vi "PDF_Interface_PDF Protokoll CalGas.vi"(8 "error in (no error)":errorcluster caption="Fehler (Eingang, kein Fehler)", 10 "Save PDF File Path":path, 11 "Zeitstempel":timestamp) -> (0 "error out":errorcluster caption="Fehler (Ausgang)")   [LabVIEW 2020, in "Erweiterte Konfig.lvlib" / "CG-Check Konfig.lvlib"]
uses:
  CG-Check Konfig.lvlib
  Sprachverwaltung/FGV Aktion Tabelle zerlegen.ctl
  System Einstellungen V2/Aktioen FGV System Konstanten.ctl
  Aktion_CG-Check.ctl
  Schedule Modul/Aktion FGV Testdaten sammeln.ctl
  FT-IR/FGV FT-IR Gasliste Aktionen.ctl
  Gaszuordnung AO/FGV Gaszuordnung Grenzen&Einheit Aktion.ctl
  PDF_Interface/PDF Protokoll Standard Kopf Optionen.ctl
  <vilib>/Simplicity AI/SAI_PDF_API/Classes/Context/Controls/SAI_PDF_PDF Details.ctl
  PDF_Interface/PDF Interface Helper/PDFContentType.ctl
  PDF_Interface/PDF Interface Helper/PDFTableContentType.ctl
  PDF_Interface/PDF Interface Helper/PDFResults.ctl
  PDF_Interface/PDF Interface Helper/PDFResultPictures.ctl
  PDF_Interface/PDF Interface Helper/PDFCommentPosition.ctl
  PDF_Interface/PDF Interface Helper/PDFPageBreak.ctl
  PDF_Interface/PDF Interface Helper/PDFTablePictures.ctl
  PDF_Interface/PDF Interface Helper/PDFBemerkung.ctl
  <vilib>/Simplicity AI/SAI_PDF_API/Classes/Context/Controls/SAI_PDF_Text Align.ctl
  <vilib>/Simplicity AI/SAI_PDF_API/Classes/Context/Controls/SAI_PDF_Font.ctl
  <vilib>/Simplicity AI/SAI_PDF_API/Classes/Context/Controls/SAI_PDF_Font Encoding.ctl
  Schedule Modul/Schedule Modul.lvlib
  System Einstellungen V2/System Einstellungen V2.lvlib
  FT-IR/FT-IR.lvlib
  Gaszuordnung AO/Gaszuordnung AO.lvlib
  Allgemein/allgemeine Sub-VIs.lvlib
  Sprachverwaltung/Sprachverwaltung.lvlib
  Linearisierung V2/Protokoll/Protokoll.lvlib
  PDF_Interface/PDF Interface.lvlib
  <vilib>/Simplicity AI/SAI_PDF_API/Classes/Context/Context.lvclass
  PDF_Interface/PDF Interface Helper/PDF Interface Helper.lvlib
panel:
  out "Span Eingang 3":string[][](table)
  out "Ergebnis 3":string caption="Auswertung:"
  out "Span Eingang 2":string[][](table)
  out "Ergebnis 2":string caption="Auswertung:"
  out "Span Eingang 1":string[][](table)
  out "Ergebnis":string caption="Auswertung:"
  out "Datum":string caption="Datum:"
  out "Messgerät:":string
  # "Kalibriergastest Protokoll"
  # "Ergebnisse:"
  # "IAG-Industrie Automatisierungsgeschellschaft m.b.H.    l  Industriestraße 322    l    2722Weikersdorf     )+43262241712/0"
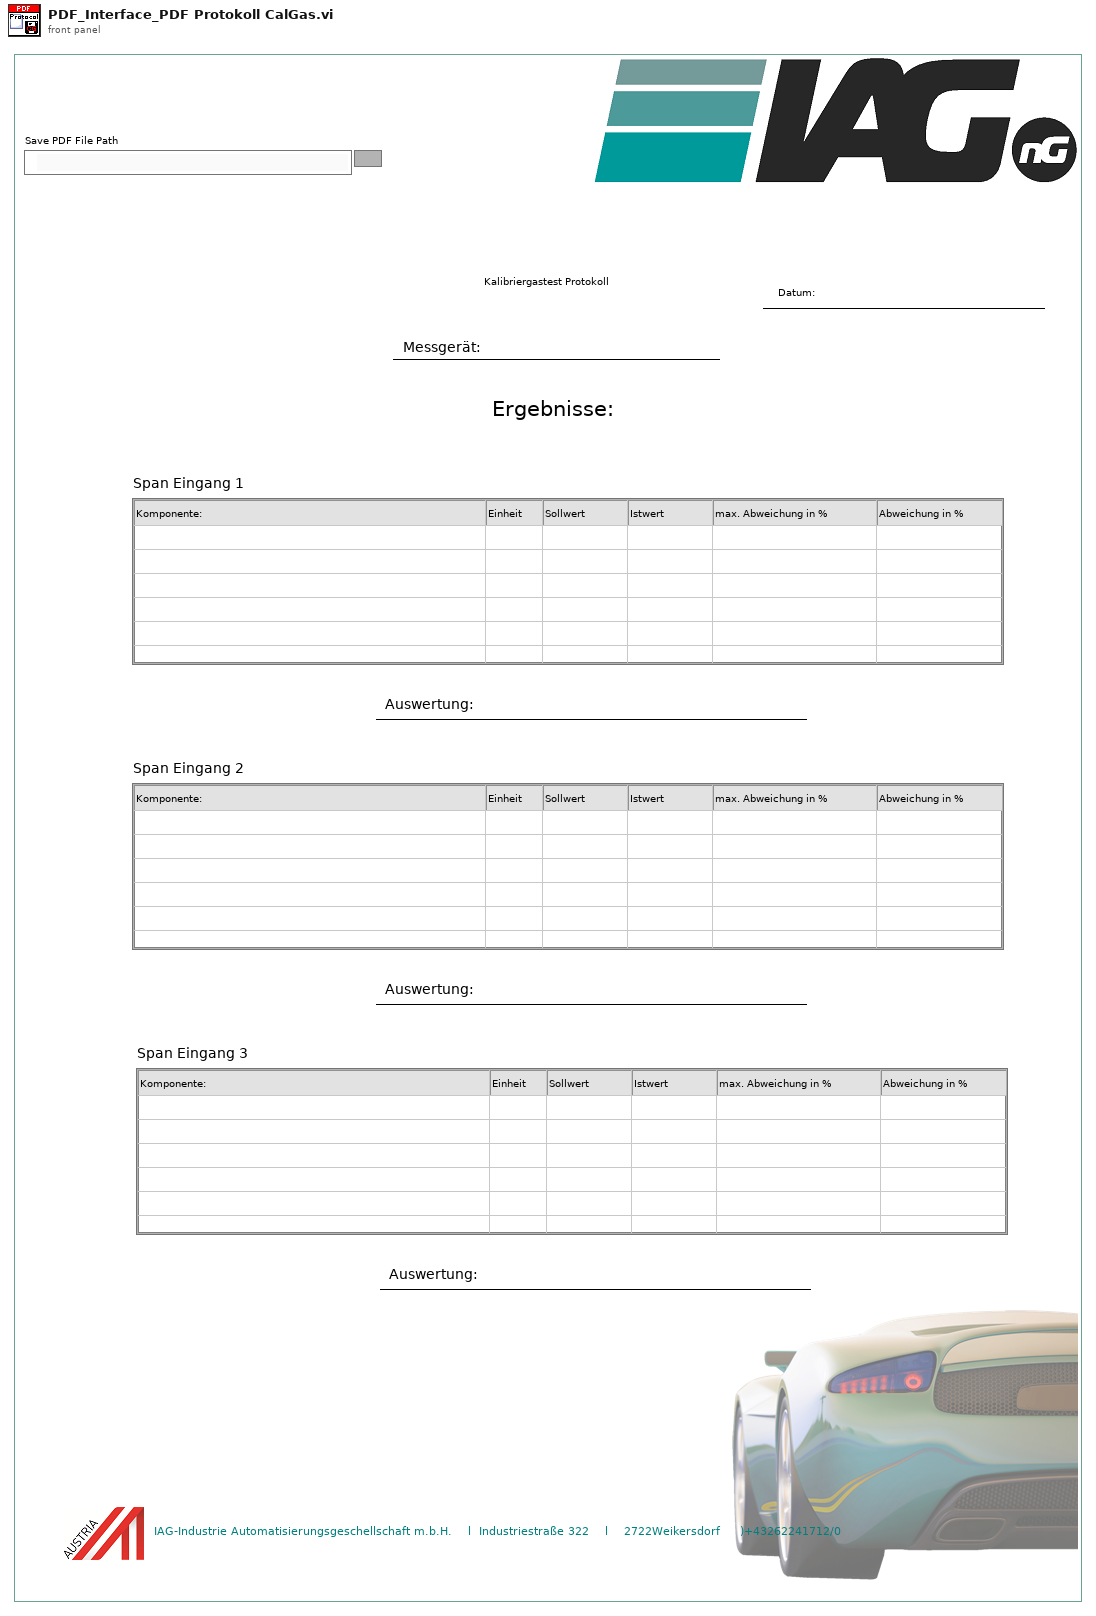
[diagram p1: front panel]
types:
  T1 = typedef "Sprachverwaltung.lvlib/FGV Aktion Tabelle zerlegen.ctl" = enum16{"laden", "vereinzeln", "speichern"}
  T2 = typedef "Schedule Modul.lvlib/Aktion FGV Testdaten sammeln.ctl" = enum16{"lesen", "Dichtheitstest", "CalGasTest", "T90", "Kalibrieren", "init", "Kalender Daten"}
  T3 = typedef "Erweiterte Konfig.lvlib/CG-Check Konfig.lvlib/Aktion_CG-Check.ctl" = enum16{"lesen", "schreiben", "laden", "Komponente", "Aktive?", "speichern"}
  T4 = typedef "System Einstellungen V2.lvlib/Aktioen FGV System Konstanten.ctl" = enum16{"lesen", "laden", "speichern", "Sprache"}
  T5 = typedef "FT-IR.lvlib/FGV FT-IR Gasliste Aktionen.ctl" = enum16{"lesen", "Gasliste FT-IR", "Gasliste ausgelesen", "laden", "speichern", "löschen"}
  T6 = typedef "Gaszuordnung AO.lvlib/FGV Gaszuordnung Grenzen&Einheit Aktion.ctl" = enum16{"Lesen", "Schreiben Min", "Schreiben Max", "Laden", "Speichern"}
  T7 = typedef "PDF Interface.lvlib/PDF Interface Helper.lvlib/PDFTableContentType.ctl" = cluster{"TableHeader":string[], "Table":string[][], "Relative Column Widths (%)":sgl[], "Results":T8, "PositionBemerkung":T10, "PageBreak":T11, "TablePictures":T12, "Horizontal Align":i32}
  T8 = typedef "PDF Interface.lvlib/PDF Interface Helper.lvlib/PDFResults.ctl" = cluster{"Results":cluster{"Result Text":string, "Result":bool}[], "ResultPictures":T9, "use Pictures":bool, "Image Scale (%)":sgl, "Autoscale? (T)":bool, "Horizontal Align":i32, "Position":i32}
  T9 = typedef "PDF Interface.lvlib/PDF Interface Helper.lvlib/PDFResultPictures.ctl" = cluster{"Yes Ctl Refnum":refnum<vi>, "No Ctl Refnum":refnum<vi>}
  T10 = typedef "PDF Interface.lvlib/PDF Interface Helper.lvlib/PDFCommentPosition.ctl" = enum16{"before", "after"}
  T11 = typedef "PDF Interface.lvlib/PDF Interface Helper.lvlib/PDFPageBreak.ctl" = enum16{"none", "before", "after", "after comment"}
  T12 = typedef "PDF Interface.lvlib/PDF Interface Helper.lvlib/PDFTablePictures.ctl" = cluster{"Ctl Refnum In":refnum<vi>[], "RowOrColumn":enum16{"Row", "Column"}, "IndexToInsert":u16, "Image Scale (%)":sgl[], "Autoscale? (T)":bool[], "Horizontal Align":i32}
  T13 = typedef "PDF Interface.lvlib/PDF Interface Helper.lvlib/PDFContentType.ctl" = cluster{"Titel":string, "Header Table":string[][], "Table Array":T7[], "Bemerkungen":T14[]}
  T14 = typedef "PDF Interface.lvlib/PDF Interface Helper.lvlib/PDFBemerkung.ctl" = cluster{"Bemerkung Text":string, "Align (Left)":T15, "Add Line Feeds (F:No)":bool, "Font":T16}
  T15 = typedef "SAI_PDF_Toolkit.lvlib/Context.lvclass/SAI_PDF_Text Align.ctl" = i32
  T16 = typedef "SAI_PDF_Toolkit.lvlib/Context.lvclass/SAI_PDF_Font.ctl" = cluster{"Font":string, "Size":i32, "Colour":u32, "Bold":bool, "Italic":bool, "Underline":bool, "Strikethrough":bool, "Font Encoding":T17}
  T17 = typedef "SAI_PDF_Toolkit.lvlib/Context.lvclass/SAI_PDF_Font Encoding.ctl" = enum16{"Cp1252, WinANSI", "IdentityH", "IdentityV", "Cp1250", "Cp1257", "MacRoman"}
  T18 = typedef "SAI_PDF_Toolkit.lvlib/Context.lvclass/SAI_PDF_PDF Details.ctl" = cluster{"Title":string, "Subject":string, "Keywords":string, "Author":string, "Creator":string}
  T19 = cluster{"Header Footer Text Cluster":cluster{"Header Text":string, "Footer Text":string, "Time":string, "Page Number":string}, "PDF Details":T18}
  T20 = typedef "PDF Interface.lvlib/PDF Protokoll Standard Kopf Optionen.ctl" = cluster{"Analysator":bool, "FT-IR Rezept":bool, "Gasteiler":bool, "Gas Komponente":bool, "Gas Flasche":bool, "LIN Protokoll":bool, "Operator":bool}
  T21 = typedef "Schedule Modul.lvlib/Ergebnis CalGas Test.ctl" = cluster{"Istwerte":string[][], "Auswertung":string[][][], "Fehler":bool[], "Abweichung in %":string[][], "Spanauswahl":i32[]}
  T22 = typedef "String - Ausgabefeld.ctl" = string
  T23 = cluster{"Modell":string, "ProjektNummer":string, "Software Version":string, "Seriennummer":string}
  T24 = cluster{"Header Size":i32, "Column Ratio left":sgl[]}
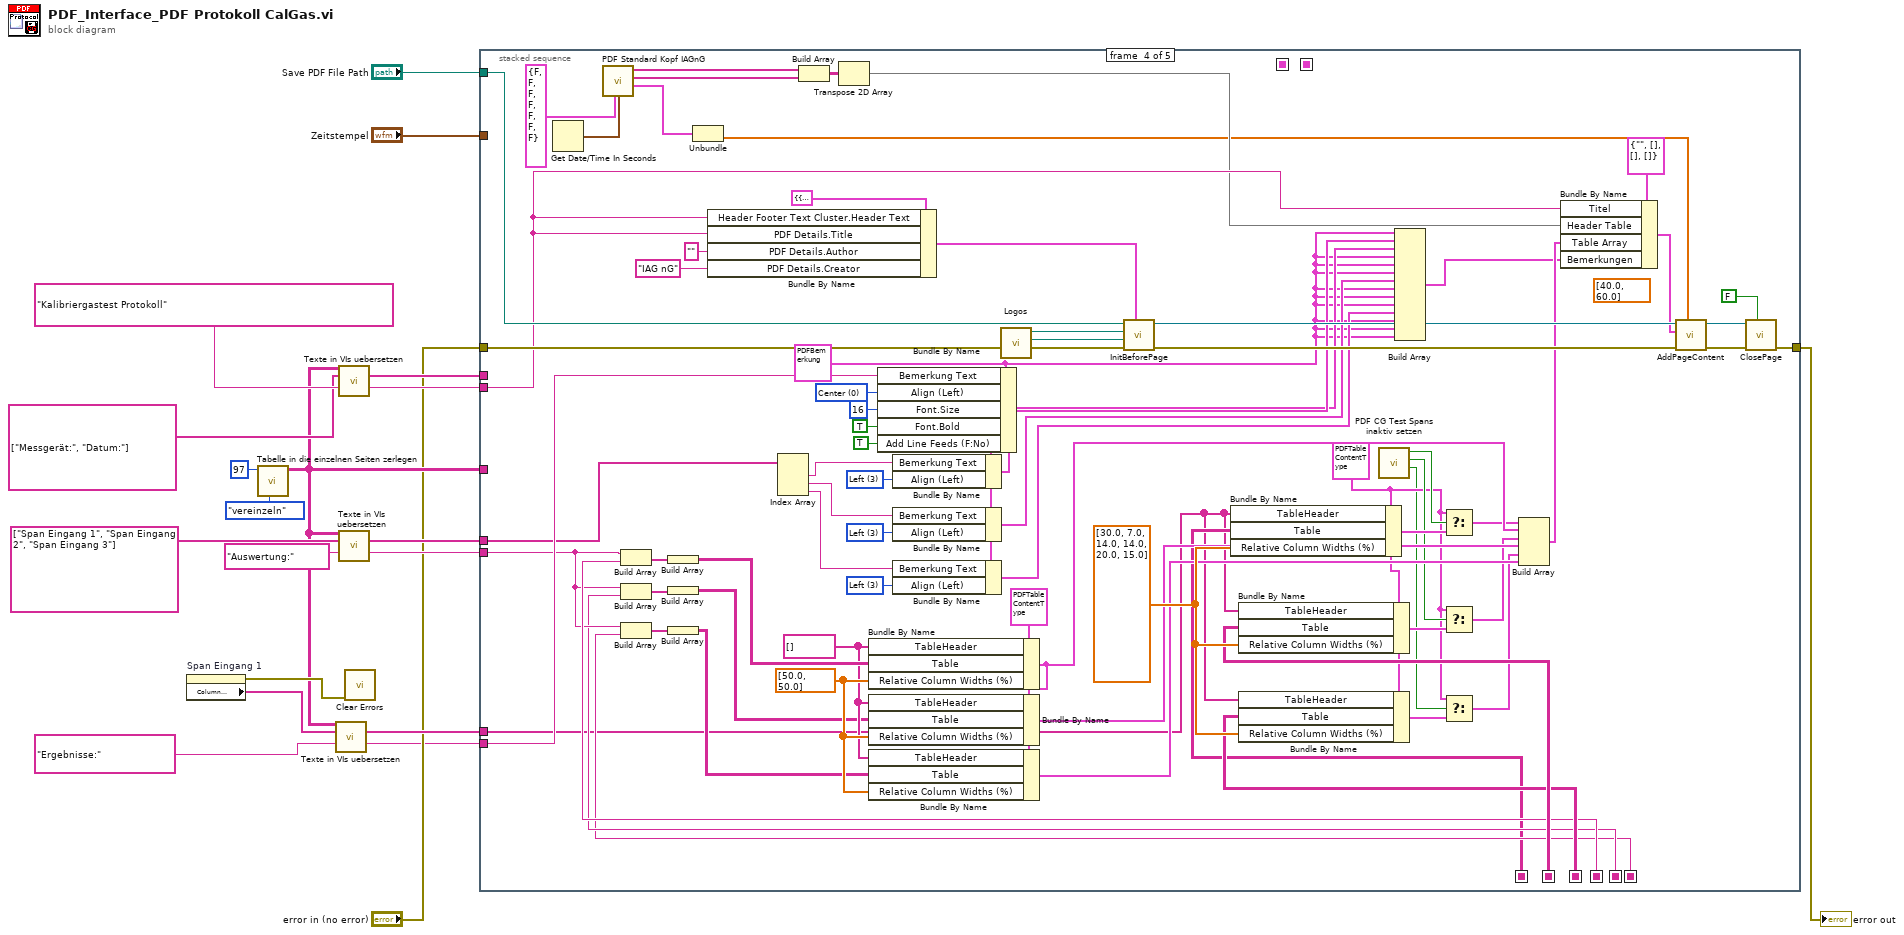
[diagram p0: block diagram]
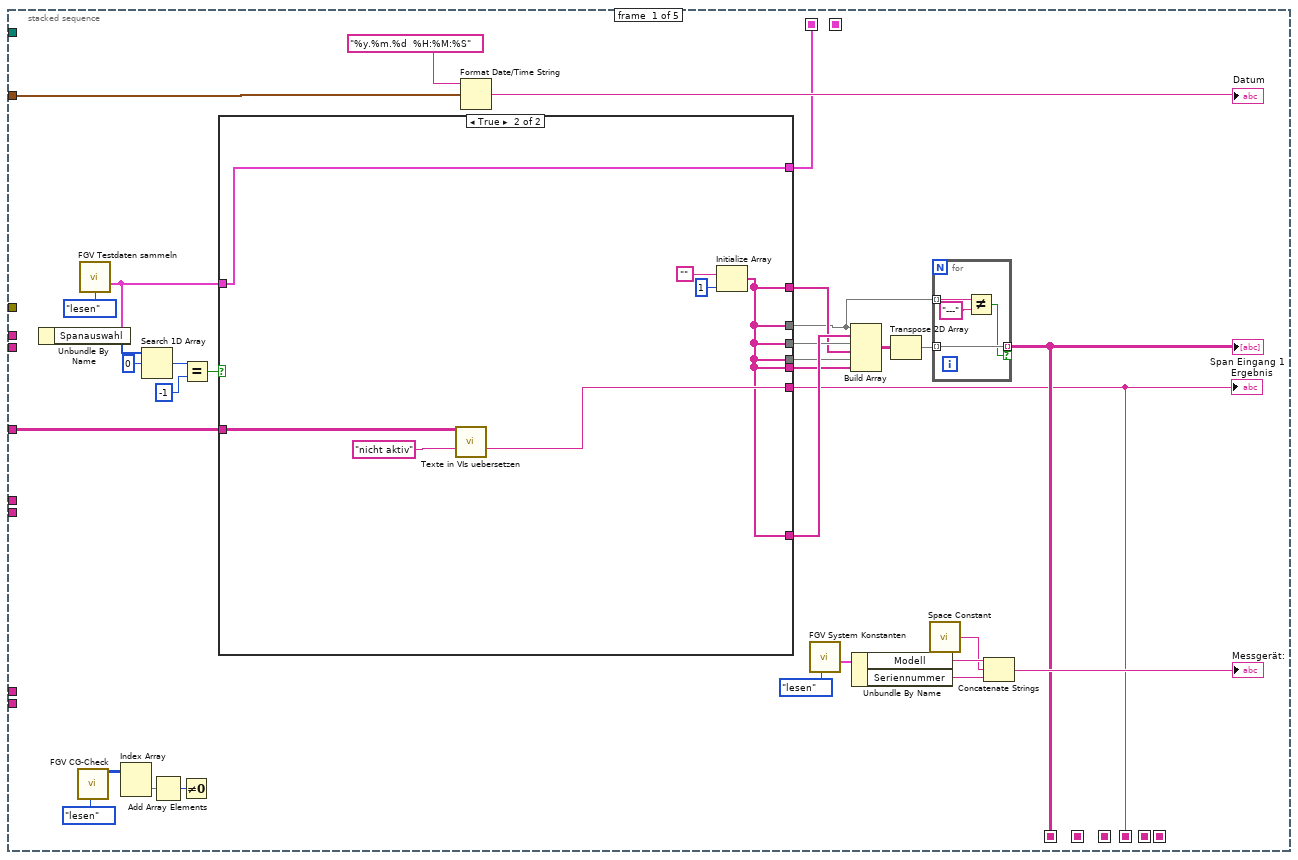
[diagram p2: hidden frame]
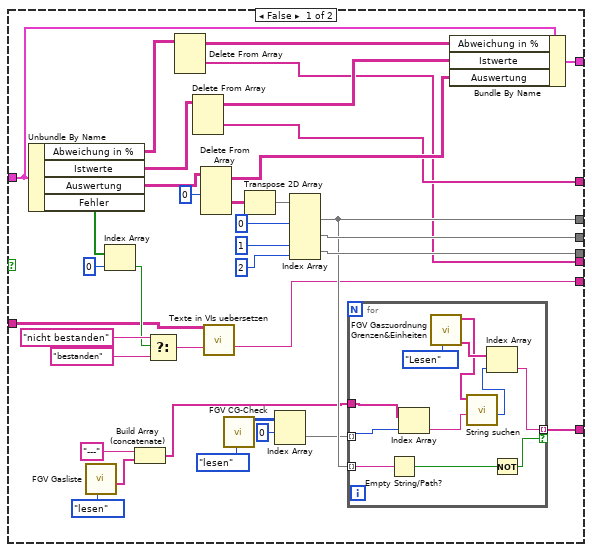
[diagram p3: hidden frame]
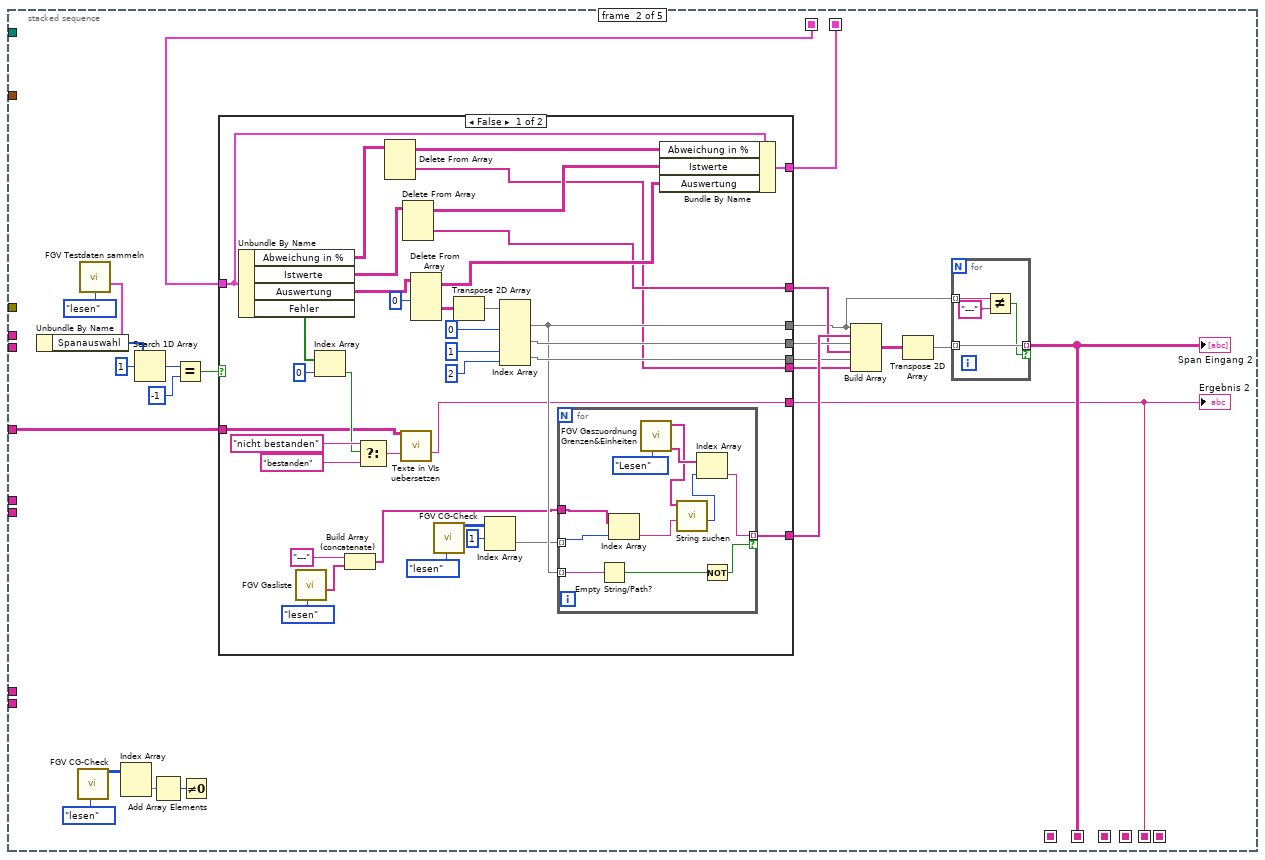
[diagram p4: hidden frame]
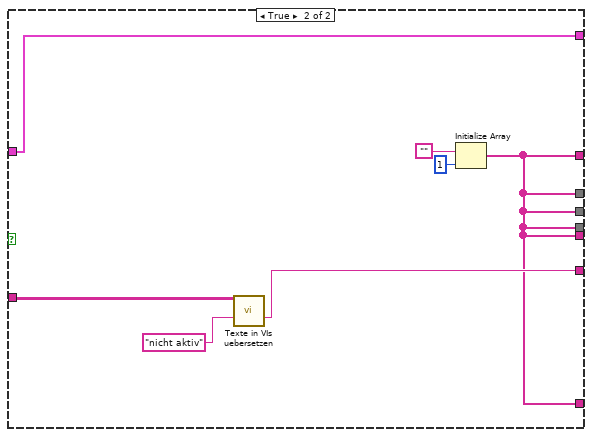
[diagram p5: hidden frame]
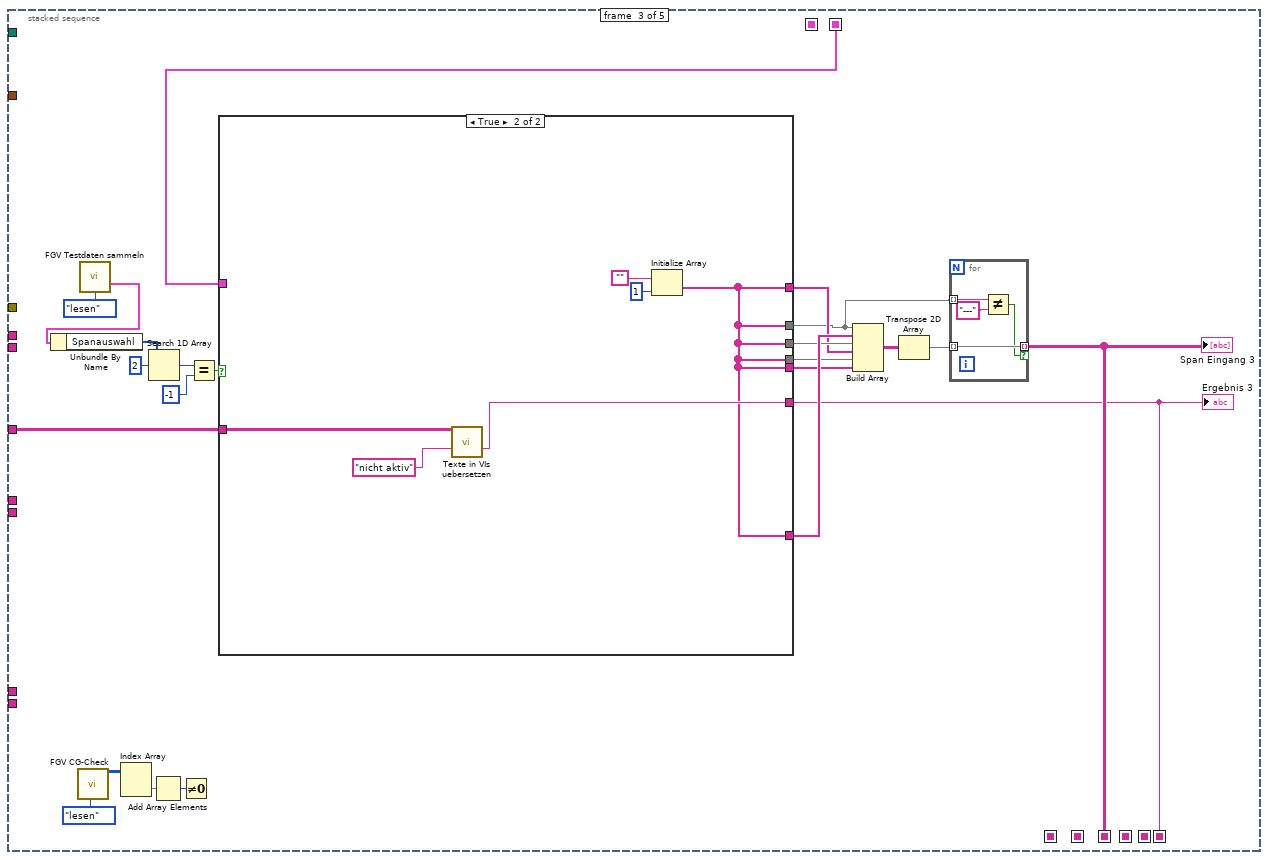
[diagram p6: hidden frame]
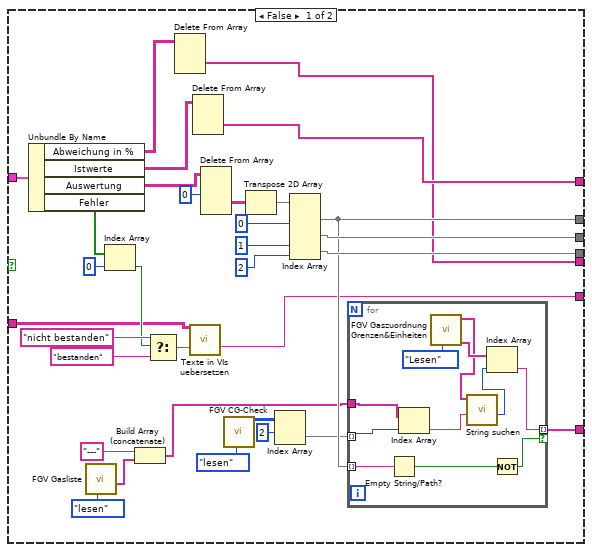
[diagram p7: hidden frame]
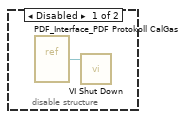
[diagram p9: hidden frame]
diagram:
  n1 = property on="Span Eingang 1" class="Tbl (strikt)"() -> (error out=w9:errorcluster, "Column Headers[]"=w8:string[])  [unwired: 2 in, 1 out]
  n2 = call "Tabelle in die einzelnen Seiten zerlegen.vi"("Aktion"=FGV_Aktion_Tabelle_zerlegen."vereinzeln", "Index (Seite)"=97) -> ("Sprachliste"=w7:string[][])  [unwired: 7 in, 2 out]
  n3 = call "Texte in VIs uebersetzen.vi"("Sprachliste"=w7, "String-Array zum Übersetzen"=w8, "String zum Übersetzen"="Ergebnisse:") -> ("String-Array zum Übersetzen"=w6:string[], "String zum Übersetzen"=w1:string)  [unwired: 8 in, 3 out]
  n4 = call "Texte in VIs uebersetzen.vi"("Sprachliste"=w7, "String-Array zum Übersetzen"=string[] ["Messgerät:", "Datum:"], "String zum Übersetzen"="Kalibriergastest Protokoll") -> ("String-Array zum Übersetzen"=w14:string[], "String zum Übersetzen"=w15:string)  [unwired: 8 in, 3 out]
  n5 = call "Texte in VIs uebersetzen.vi"("Sprachliste"=w7, "String-Array zum Übersetzen"=string[] ["Span Eingang 1", "Span Eingang 2", "Span Eingang 3"], "String zum Übersetzen"="Auswertung:") -> ("String-Array zum Übersetzen"=w12:string[], "String zum Übersetzen"=w10:string)  [unwired: 8 in, 3 out]
  n6 = call <vilib>:"Clear Errors.vi"("error in (no error)"=w9) -> ()  [unwired: 5 in, 2 out]
  n7 = stacked-sequence {
    seq-local: [w32 _ _ _ _] -> [_ w122 _ _ _]
    seq-local: [_ w121 _ _ _] -> [_ _ w205 _ _]
    seq-local: [w22 _ _ _ _] -> [_ _ _ w280 _]
    seq-local: [_ w112 _ _ _] -> [_ _ _ w322 _]
    seq-local: [_ _ w194 _ _] -> [_ _ _ w321 _]
    seq-local: [w21 _ _ _ _] -> [_ _ _ w298 _]
    seq-local: [_ w111 _ _ _] -> [_ _ _ w296 _]
    seq-local: [_ _ w193 _ _] -> [_ _ _ w295 _]
    tunnel: w7 -> [w24 w113 w195 _ _]
    tunnel: "Save PDF File Path" -> [_ _ _ w328 _]
    tunnel: w15 -> [_ _ _ w325 _]
    tunnel: w14 -> [_ _ _ _ _]
    tunnel: w12 -> [_ _ _ w307 _]
    tunnel: w10 -> [_ _ _ w297 _]
    tunnel: w6 -> [_ _ _ w279 _]
    tunnel: "Zeitstempel" -> [w23 _ _ _ _]
    tunnel: "error in (no error)" -> [_ _ _ w327 _]
    tunnel: [_ _ _ w326 _] -> w3
    tunnel: w1 -> [_ _ _ w313 _]
    frame #0 {
      n8 = call "FGV CG-Check.vi"("Aktion"=Aktion_CG-Check."lesen") -> ("Komponenten"=w36:u16[][])  [unwired: 11 in, 7 out]
      n9 = call "FGV Testdaten sammeln.vi"("Aktion"=Aktion_FGV_Testdaten_sammeln."lesen") -> ("Ergebnis CalGas Test"=w34:T21)  [unwired: 9 in, 5 out]
      n10 = Unbundle By Name(w34) -> ("Spanauswahl"=w31:i32[])
      n11 = Index Array(array=w36) -> (element=w38:u16[])  [unwired: 2 in]
      n12 = Search 1D Array(1D array=w31, element=0 ("Element")) -> (index of element=w29:i32)  [unwired: 1 in]
      n13 = Add Array Elements(numeric array=w38) -> (sum=w39:u16)
      n14 = Not Equal To 0?(x=w39) -> ()  [unwired: 1 out]
      n15 = Equal?(x=w29, y=-1) -> (x = y?=w33:bool)
      n16 = case shown="True" w33 {
        tunnel: [w79 w104] -> w25
        tunnel: [w78 w104] -> w44
        tunnel: [w89 w104] -> w43
        tunnel: [w64 w104] -> w42
        tunnel: [w88 w104] -> w41
        tunnel: [w63 w104] -> w40
        tunnel: w34 -> [w71 w110]
        tunnel: [w62 w110] -> w32
        tunnel: w24 -> [w58 w108]
        tunnel: [w57 w107] -> w21
        frame False {
          n17 = Unbundle By Name(w71) -> ("Abweichung in %"=w87:string[][], "Istwerte"=w69:string[][], "Auswertung"=w67:string[][][], "Fehler"=w84:bool[])
          n18 = call "FGV Gasliste.vi"("Aktionen"=FGV_FT-IR_Gasliste_Aktionen."lesen") -> ("Aktuelle Gasliste gesamt"=w74:T22[])  [unwired: 8 in, 2 out]
          n19 = Index Array(array=w84, index=0 ("Index")) -> (element=w82:bool)
          n20 = Build Array (concatenate)("---", w74) -> (w73:T22[])
          n21 = Select(t="nicht bestanden" ("String"), s=w82, f="bestanden" ("String")) -> (s? t:f=w59:string)
          n22 = Delete From Array(array=w87) -> (deleted portion=w63:string[], array with subset deleted=w70:string[][])  [unwired: 3 in]
          n23 = Delete From Array(array=w69) -> (deleted portion=w64:string[], array with subset deleted=w68:string[][])  [unwired: 3 in]
          n24 = Delete From Array(array=w67, index (dim 0)=0 ("Index (Seite)")) -> (deleted portion=w65:string[][], array with subset deleted=w66:string[][][])  [unwired: 3 in]
          n25 = call "Texte in VIs uebersetzen.vi"("Sprachliste"=w58, "String zum Übersetzen"=w59) -> ("String zum Übersetzen"=w57:string)  [unwired: 9 in, 4 out]
          n26 = call "FGV CG-Check.vi"("Aktion"=Aktion_CG-Check."lesen") -> ("Komponenten"=w80:u16[][])  [unwired: 11 in, 7 out]
          n27 = Transpose 2D Array(2D array=w65) -> (transposed array=w60:string[][])
          n28 = Index Array(array=w80, index (row)=0 ("Index (Zeile)")) -> (element=w72:u16[])  [unwired: 1 in]
          n29 = Index Array(array=w60, index (col) #1=0 ("Deaktivierter Index (Zeile)"), index (col) #2=1 ("Deaktivierter Index (Zeile)"), index (col) #3=2 ("Deaktivierter Index (Zeile)")) -> (element #1=w79:string[], element #2=w89:string[], element #3=w88:string[])  [unwired: 3 in]
          n30 = for {
            tunnel: w79 -> [w98] mode=indexing
            tunnel: [w101] -> w78 mode=indexing if=w99
            tunnel: w73 -> [w97]
            tunnel: w72 -> [w96] mode=indexing
            n31 = Empty String/Path?(string/path=w98) -> (empty?=w100:bool)
            n32 = Index Array(array=w97, index=w96) -> (element=w94:T22)
            n33 = call "FGV Gaszuordnung Grenzen&Einheiten.vi"("Aktion"=FGV_Gaszuordnung_Grenzen&Einheit_Aktion."Lesen") -> ("Einheit neu"=w102:string[], "Namen neu"=w95:string[])  [unwired: 7 in, 2 out]
            n34 = call "String suchen.vi"("Gasname"=w94, "Such-Namen"=w95) -> ("Index"=w93:i32)  [unwired: 8 in, 1 out]
            n35 = Index Array(array=w102, index=w93) -> (element=w101:string)
            n36 = Not(x=w100) -> (.not. x?=w99:bool)
          }
          n37 = Bundle By Name(cluster=w71, "Abweichung in %"=w70, "Istwerte"=w68, "Auswertung"=w66) -> (w62:T21)
        }
        frame True {
          n38 = call "Texte in VIs uebersetzen.vi"("Sprachliste"=w108, "String zum Übersetzen"="nicht aktiv" ("f")) -> ("String zum Übersetzen"=w107:string)  [unwired: 9 in, 4 out]
          n39 = Initialize Array("", 1 ("Dimensionsgröße")) -> (w104:string[])
        }
      }
      "Ergebnis" <- w21
      n40 = Format Date/Time String(time format string (%c)="%y.%m.%d  %H:%M:%S" ("Zeitformatierungs-String (%c)"), seconds (now)=w23) -> (date/time string=→"Datum":string)  [unwired: 1 in]
      n41 = call "FGV System Konstanten.vi"("Aktionen"=Aktioen_FGV_System_Konstanten."lesen") -> ("Cluster out"=w51:T23)  [unwired: 6 in, 4 out]
      n42 = Build Array(w25, w44, w43, w42, w41, w40) -> (w27:string[][])
      n43 = Unbundle By Name(w51) -> ("Modell"=w50:string, "Seriennummer"=w48:string)
      n44 = Transpose 2D Array(2D array=w27) -> (transposed array=w26:string[][])
      n45 = call <vilib>:"Space Constant.vi"() -> ("String"=w49:string)
      n46 = for {
        tunnel: [w56] -> w22 mode=indexing if=w53
        tunnel: w26 -> [w56] mode=indexing
        tunnel: w25 -> [w55] mode=indexing
        n47 = Not Equal?(x=w55, y="---") -> (x != y?=w53:bool)
      }
      "Span Eingang 1" <- w22
      n48 = Concatenate Strings(w50, w49, w48) -> (→"Messgerät:":string)
    }
    frame #1 {
      n49 = call "FGV CG-Check.vi"("Aktion"=Aktion_CG-Check."lesen") -> ("Komponenten"=w126:u16[][])  [unwired: 11 in, 7 out]
      n50 = call "FGV Testdaten sammeln.vi"("Aktion"=Aktion_FGV_Testdaten_sammeln."lesen") -> ("Ergebnis CalGas Test"=w124:T21)  [unwired: 9 in, 5 out]
      n51 = Unbundle By Name(w124) -> ("Spanauswahl"=w119:i32[])
      n52 = Index Array(array=w126) -> (element=w128:u16[])  [unwired: 2 in]
      n53 = Search 1D Array(1D array=w119, element=1 ("Element")) -> (index of element=w118:i32)  [unwired: 1 in]
      n54 = Add Array Elements(numeric array=w128) -> (sum=w129:u16)
      n55 = Equal?(x=w118, y=-1) -> (x = y?=w123:bool)
      n56 = Not Equal To 0?(x=w129) -> ()  [unwired: 1 out]
      n57 = case shown="False" w123 {
        tunnel: [w161 w186] -> w114
        tunnel: [w160 w186] -> w134
        tunnel: [w171 w186] -> w133
        tunnel: [w146 w186] -> w132
        tunnel: [w170 w186] -> w131
        tunnel: [w145 w186] -> w130
        tunnel: w122 -> [w153 w192]
        tunnel: [w144 w192] -> w121
        tunnel: w113 -> [w140 w190]
        tunnel: [w139 w189] -> w111
        frame False {
          n58 = Unbundle By Name(w153) -> ("Abweichung in %"=w169:string[][], "Istwerte"=w151:string[][], "Auswertung"=w149:string[][][], "Fehler"=w166:bool[])
          n59 = call "FGV Gasliste.vi"("Aktionen"=FGV_FT-IR_Gasliste_Aktionen."lesen") -> ("Aktuelle Gasliste gesamt"=w156:T22[])  [unwired: 8 in, 2 out]
          n60 = Index Array(array=w166, index=0 ("Index")) -> (element=w164:bool)
          n61 = Build Array (concatenate)("---", w156) -> (w155:T22[])
          n62 = Select(t="nicht bestanden" ("String"), s=w164, f="bestanden" ("String")) -> (s? t:f=w141:string)
          n63 = Delete From Array(array=w169) -> (deleted portion=w145:string[], array with subset deleted=w152:string[][])  [unwired: 3 in]
          n64 = call "Texte in VIs uebersetzen.vi"("Sprachliste"=w140, "String zum Übersetzen"=w141) -> ("String zum Übersetzen"=w139:string)  [unwired: 9 in, 4 out]
          n65 = Delete From Array(array=w151) -> (deleted portion=w146:string[], array with subset deleted=w150:string[][])  [unwired: 3 in]
          n66 = Delete From Array(array=w149, index (dim 0)=0 ("Index (Seite)")) -> (deleted portion=w147:string[][], array with subset deleted=w148:string[][][])  [unwired: 3 in]
          n67 = call "FGV CG-Check.vi"("Aktion"=Aktion_CG-Check."lesen") -> ("Komponenten"=w162:u16[][])  [unwired: 11 in, 7 out]
          n68 = Transpose 2D Array(2D array=w147) -> (transposed array=w142:string[][])
          n69 = Index Array(array=w162, index (row)=1 ("Index (Zeile)")) -> (element=w154:u16[])  [unwired: 1 in]
          n70 = Index Array(array=w142, index (col) #1=0 ("Deaktivierter Index (Zeile)"), index (col) #2=1 ("Deaktivierter Index (Zeile)"), index (col) #3=2 ("Deaktivierter Index (Zeile)")) -> (element #1=w161:string[], element #2=w171:string[], element #3=w170:string[])  [unwired: 3 in]
          n71 = for {
            tunnel: w161 -> [w180] mode=indexing
            tunnel: [w183] -> w160 mode=indexing if=w181
            tunnel: w155 -> [w179]
            tunnel: w154 -> [w178] mode=indexing
            n72 = Empty String/Path?(string/path=w180) -> (empty?=w182:bool)
            n73 = Index Array(array=w179, index=w178) -> (element=w176:T22)
            n74 = call "FGV Gaszuordnung Grenzen&Einheiten.vi"("Aktion"=FGV_Gaszuordnung_Grenzen&Einheit_Aktion."Lesen") -> ("Einheit neu"=w184:string[], "Namen neu"=w177:string[])  [unwired: 7 in, 2 out]
            n75 = call "String suchen.vi"("Gasname"=w176, "Such-Namen"=w177) -> ("Index"=w175:i32)  [unwired: 8 in, 1 out]
            n76 = Index Array(array=w184, index=w175) -> (element=w183:string)
            n77 = Not(x=w182) -> (.not. x?=w181:bool)
          }
          n78 = Bundle By Name(cluster=w153, "Abweichung in %"=w152, "Istwerte"=w150, "Auswertung"=w148) -> (w144:T21)
        }
        frame True {
          n79 = call "Texte in VIs uebersetzen.vi"("Sprachliste"=w190, "String zum Übersetzen"="nicht aktiv" ("f")) -> ("String zum Übersetzen"=w189:string)  [unwired: 9 in, 4 out]
          n80 = Initialize Array("", 1 ("Dimensionsgröße")) -> (w186:string[])
        }
      }
      "Ergebnis 2" <- w111
      n81 = Build Array(w114, w134, w133, w132, w131, w130) -> (w116:string[][])
      n82 = Transpose 2D Array(2D array=w116) -> (transposed array=w115:string[][])
      n83 = for {
        tunnel: [w138] -> w112 mode=indexing if=w135
        tunnel: w115 -> [w138] mode=indexing
        tunnel: w114 -> [w137] mode=indexing
        n84 = Not Equal?(x=w137, y="---") -> (x != y?=w135:bool)
      }
      "Span Eingang 2" <- w112
    }
    frame #2 {
      n85 = call "FGV CG-Check.vi"("Aktion"=Aktion_CG-Check."lesen") -> ("Komponenten"=w207:u16[][])  [unwired: 11 in, 7 out]
      n86 = call "FGV Testdaten sammeln.vi"("Aktion"=Aktion_FGV_Testdaten_sammeln."lesen") -> ("Ergebnis CalGas Test"=w200:T21)  [unwired: 9 in, 5 out]
      n87 = Unbundle By Name(w200) -> ("Spanauswahl"=w201:i32[])
      n88 = Index Array(array=w207) -> (element=w209:u16[])  [unwired: 2 in]
      n89 = Search 1D Array(1D array=w201, element=2 ("Element")) -> (index of element=w203:i32)  [unwired: 1 in]
      n90 = Add Array Elements(numeric array=w209) -> (sum=w210:u16)
      n91 = Not Equal To 0?(x=w210) -> ()  [unwired: 1 out]
      n92 = Equal?(x=w203, y=-1) -> (x = y?=w199:bool)
      n93 = case shown="True" w199 {
        tunnel: [w238 w263] -> w196
        tunnel: [w237 w263] -> w215
        tunnel: [w248 w263] -> w214
        tunnel: [w226 w263] -> w213
        tunnel: [w247 w263] -> w212
        tunnel: [w225 w263] -> w211
        tunnel: w205 -> [w230 _]
        tunnel: w195 -> [w221 w267]
        tunnel: [w220 w266] -> w193
        frame False {
          n94 = Unbundle By Name(w230) -> ("Abweichung in %"=w246:string[][], "Istwerte"=w229:string[][], "Auswertung"=w228:string[][][], "Fehler"=w243:bool[])
          n95 = call "FGV Gasliste.vi"("Aktionen"=FGV_FT-IR_Gasliste_Aktionen."lesen") -> ("Aktuelle Gasliste gesamt"=w233:T22[])  [unwired: 8 in, 2 out]
          n96 = Index Array(array=w243, index=0 ("Index")) -> (element=w241:bool)
          n97 = Build Array (concatenate)("---", w233) -> (w232:T22[])
          n98 = Select(t="nicht bestanden" ("String"), s=w241, f="bestanden" ("String")) -> (s? t:f=w222:string)
          n99 = Delete From Array(array=w246) -> (deleted portion=w225:string[])  [unwired: 3 in, 1 out]
          n100 = call "Texte in VIs uebersetzen.vi"("Sprachliste"=w221, "String zum Übersetzen"=w222) -> ("String zum Übersetzen"=w220:string)  [unwired: 9 in, 4 out]
          n101 = Delete From Array(array=w229) -> (deleted portion=w226:string[])  [unwired: 3 in, 1 out]
          n102 = Delete From Array(array=w228, index (dim 0)=0 ("Index (Seite)")) -> (deleted portion=w227:string[][])  [unwired: 3 in, 1 out]
          n103 = call "FGV CG-Check.vi"("Aktion"=Aktion_CG-Check."lesen") -> ("Komponenten"=w239:u16[][])  [unwired: 11 in, 7 out]
          n104 = Transpose 2D Array(2D array=w227) -> (transposed array=w223:string[][])
          n105 = Index Array(array=w239, index (row)=2 ("Index (Zeile)")) -> (element=w231:u16[])  [unwired: 1 in]
          n106 = Index Array(array=w223, index (col) #1=0 ("Deaktivierter Index (Zeile)"), index (col) #2=1 ("Deaktivierter Index (Zeile)"), index (col) #3=2 ("Deaktivierter Index (Zeile)")) -> (element #1=w238:string[], element #2=w248:string[], element #3=w247:string[])  [unwired: 3 in]
          n107 = for {
            tunnel: w238 -> [w257] mode=indexing
            tunnel: [w260] -> w237 mode=indexing if=w258
            tunnel: w232 -> [w256]
            tunnel: w231 -> [w255] mode=indexing
            n108 = Empty String/Path?(string/path=w257) -> (empty?=w259:bool)
            n109 = Index Array(array=w256, index=w255) -> (element=w253:T22)
            n110 = call "FGV Gaszuordnung Grenzen&Einheiten.vi"("Aktion"=FGV_Gaszuordnung_Grenzen&Einheit_Aktion."Lesen") -> ("Einheit neu"=w261:string[], "Namen neu"=w254:string[])  [unwired: 7 in, 2 out]
            n111 = call "String suchen.vi"("Gasname"=w253, "Such-Namen"=w254) -> ("Index"=w252:i32)  [unwired: 8 in, 1 out]
            n112 = Index Array(array=w261, index=w252) -> (element=w260:string)
            n113 = Not(x=w259) -> (.not. x?=w258:bool)
          }
        }
        frame True {
          n114 = call "Texte in VIs uebersetzen.vi"("Sprachliste"=w267, "String zum Übersetzen"="nicht aktiv" ("f")) -> ("String zum Übersetzen"=w266:string)  [unwired: 9 in, 4 out]
          n115 = Initialize Array("", 1 ("Dimensionsgröße")) -> (w263:string[])
        }
      }
      "Ergebnis 3" <- w193
      n116 = Build Array(w196, w215, w214, w213, w212, w211) -> (w198:string[][])
      n117 = Transpose 2D Array(2D array=w198) -> (transposed array=w197:string[][])
      n118 = for {
        tunnel: [w219] -> w194 mode=indexing if=w216
        tunnel: w197 -> [w219] mode=indexing
        tunnel: w196 -> [w218] mode=indexing
        n119 = Not Equal?(x=w218, y="---") -> (x != y?=w216:bool)
      }
      "Span Eingang 3" <- w194
    }
    frame #3 {
      w290 = sgl[] [50.0, 50.0] ("Relative Column Widths (%)")
      w289 = string[] [] ("TableHeader")
      w306 = T15 3 items=["Center", "Justified", "Justified All", "Left", "Right"] ("Align (Left)")
      w309 = T15 3 items=["Center", "Justified", "Justified All", "Left", "Right"] ("Align (Left)")
      w310 = T15 3 items=["Center", "Justified", "Justified All", "Left", "Right"] ("Align (Left)")
      w314 = T15 0 items=["Center", "Justified", "Justified All", "Left", "Right"] ("Align (Left)")
      w323 = sgl[] [30.0, 7.0, 14.0, 14.0, 20.0, 15.0] ("Relative Column Widths (%)")
      w271 = T7 {"TableHeader"=[], "Table"=[], "Relative Column Widths (%)"=[], "Results"={"Results"=[], "ResultPictures"={"Yes Ctl Refnum"=refnum, "No Ctl Refnum"=refnum}, "use Pictures"=FALSE, "Image Scale (%)"=0.0, "Autoscale? (T)"=FALSE, "Horizontal Align"=0, "Position"=0}, "PositionBemerkung"=enum."before", "PageBreak"=enum."none", "TablePictures"={"Ctl Refnum In"=[], "RowOrColumn"=enum."Row", "IndexToInsert"=0, "Image Scale (%)"=[], "Autoscale? (T)"=[], "Horizontal Align"=0}, "Horizontal Align"=0} ("Table Array")
      w300 = T14 {"Bemerkung Text"="", "Align (Left)"=0, "Add Line Feeds (F:No)"=FALSE, "Font"={"Font"="Arial", "Size"=10, "Colour"=0, "Bold"=FALSE, "Italic"=FALSE, "Underline"=FALSE, "Strikethrough"=FALSE, "Font Encoding"=enum."Cp1252, WinANSI"}} ("Bemerkung")
      (unwired) sgl[] [40.0, 60.0] ("Column Ratio left")
      n120 = Get Date/Time In Seconds() -> (seconds since 1Jan1904=w343:timestamp)
      n121 = call "PDF Standard Kopf IAGnG.vi"("Zeitstempel"=w343, "Oprtionen Cluster"=T20 {"Analysator"=FALSE, "FT-IR Rezept"=FALSE, "Gasteiler"=FALSE, "Gas Komponente"=FALSE, "Gas Flasche"=FALSE, "LIN Protokoll"=FALSE, "Operator"=FALSE}) -> ("Size Cluster"=w282:T24, "Header Values"=w318:T22[], "Header Labels"=w319:string[])  [unwired: 6 in, 1 out]
      n122 = Build Array(w297, w298) -> (w294:string[])
      n123 = Build Array(w297, w296) -> (w293:string[])
      n124 = Build Array(w297, w295) -> (w292:string[])
      n125 = Build Array(w294) -> (w291:string[][])
      n126 = Build Array(w293) -> (w288:string[][])
      n127 = Build Array(w292) -> (w287:string[][])
      n128 = Unbundle(w282) -> ("Column Ratio left"=w281:sgl[])  [unwired: 1 out]
      n129 = Bundle By Name(cluster=T19 {"Header Footer Text Cluster"={"Header Text"="Protokoll XYZ", "Footer Text"="IAG nG", "Time"="<TIMESTAMP yyyy-MM-dd>", "Page Number"="Page <P> of <PT>"}, "PDF Details"={"Title"="Test PDF", "Subject"="Versa Tabasco", "Keywords"="", "Author"="RIW", "Creator"="IAG"}} ("Info"), "Header Footer Text Cluster.Header Text"=w325, "PDF Details.Title"=w325, "PDF Details.Author"="", "PDF Details.Creator"="IAG nG") -> (w331:T19)
      n130 = Index Array(array=w307) -> (element #1=w305:string, element #2=w304:string, element #3=w303:string)  [unwired: 3 in]
      n131 = Build Array(w319, w318) -> (w320:T22[][])
      n132 = Transpose 2D Array(2D array=w320) -> (transposed array=w317:T22[][])
      n133 = Bundle By Name(cluster=T7 {"TableHeader"=[], "Table"=[], "Relative Column Widths (%)"=[], "Results"={"Results"=[], "ResultPictures"={"Yes Ctl Refnum"=refnum, "No Ctl Refnum"=refnum}, "use Pictures"=FALSE, "Image Scale (%)"=0.0, "Autoscale? (T)"=FALSE, "Horizontal Align"=0, "Position"=0}, "PositionBemerkung"=enum."before", "PageBreak"=enum."none", "TablePictures"={"Ctl Refnum In"=[], "RowOrColumn"=enum."Row", "IndexToInsert"=0, "Image Scale (%)"=[], "Autoscale? (T)"=[], "Horizontal Align"=0}, "Horizontal Align"=0} ("Table Array"), "TableHeader"=w289, "Table"=w291, "Relative Column Widths (%)"=w290) -> (w284:T7)
      n134 = Bundle By Name(cluster=w284, "TableHeader"=w289, "Table"=w288, "Relative Column Widths (%)"=w290) -> (w286:T7)
      n135 = Bundle By Name(cluster=w284, "TableHeader"=w289, "Table"=w287, "Relative Column Widths (%)"=w290) -> (w285:T7)
      n136 = Bundle By Name(cluster=w300, "Bemerkung Text"=w313, "Align (Left)"=w314, "Font.Size"=16, "Font.Bold"=TRUE, "Add Line Feeds (F:No)"=TRUE) -> (w311:T14)
      n137 = Bundle By Name(cluster=w300, "Bemerkung Text"=w305, "Align (Left)"=w310) -> (w308:T14)
      n138 = Bundle By Name(cluster=w300, "Bemerkung Text"=w304, "Align (Left)"=w309) -> (w302:T14)
      n139 = Bundle By Name(cluster=w300, "Bemerkung Text"=w303, "Align (Left)"=w306) -> (w301:T14)
      n140 = call "Logos.vi"() -> ("Footer Image File Path"=w340:path, "Header Image File Path"=w341:path)  [unwired: 8 in, 2 out]
      n141 = call "InitBeforePage.vi"("Info"=w331, "Fehler (Eingang, kein Fehler)"=w327, "Footer Image File Path"=w340, "Header Image File Path"=w341, "Path (Dialog if Empty)"=w328) -> ("Fehler (Ausgang)"=w339:errorcluster, "Context (Ausgang)"=w338:refnum<class "Context.lvclass">)  [unwired: 5 in]
      n142 = Bundle By Name(cluster=w271, "TableHeader"=w279, "Table"=w280, "Relative Column Widths (%)"=w323) -> (w278:T7)
      n143 = Bundle By Name(cluster=w271, "TableHeader"=w279, "Table"=w322, "Relative Column Widths (%)"=w323) -> (w275:T7)
      n144 = Bundle By Name(cluster=w271, "TableHeader"=w279, "Table"=w321, "Relative Column Widths (%)"=w323) -> (w272:T7)
      n145 = call "PDF CG Test Spans inaktiv setzen.vi"() -> ("Span 3"=w270:bool, "Span 2"=w274:bool, "Span 1"=w276:bool)  [unwired: 9 in]
      n146 = Build Array(w300, w311, w308, w300, w300, w300, w302, w300, w300, w300, w301, w300, w300, w300) -> (w312:T14[])
      n147 = Select(t=w271, s=w276, f=w278) -> (s? t:f=w277:T7)
      n148 = Select(t=w271, s=w274, f=w275) -> (s? t:f=w273:T7)
      n149 = Select(t=w271, s=w270, f=w272) -> (s? t:f=w269:T7)
      n150 = Build Array(w277, w284, w273, w286, w269, w285) -> (w324:T7[])
      n151 = Bundle By Name(cluster=T13 {"Titel"="", "Header Table"=[], "Table Array"=[], "Bemerkungen"=[]} ("Content"), "Titel"=w325, "Header Table"=w317, "Table Array"=w324, "Bemerkungen"=w312) -> (w329:T13)
      n152 = call "AddPageContent.vi"("Column Ratio left"=w281, "error in"=w339, "Content"=w329, "Context (Eingang)"=w338) -> ("error out"=w337:errorcluster, "Context (Ausgang)"=w336:refnum<class "Context.lvclass">)  [unwired: 6 in]
      n153 = call "ClosePage.vi"("popup viewer"=FALSE, "Fehler (Eingang, kein Fehler)"=w337, "Context (Eingang)"=w336) -> ("Fehler (Ausgang)"=w326:errorcluster)  [unwired: 8 in]
    }
    frame #4 {
      n154 = disable-structure shown="Aktiviert" {
        frame Disabled {
          n155 = vi-ref "PDF_Interface_PDF Protokoll CalGas.vi"() -> (w344:refnum<vi>)
          n156 = call "VI Shut Down.vi"("VI Referenz"=w344) -> ()  [unwired: 11 in]
        }
        frame Enabled {
        }
      }
    }
  }
  "error out" <- w3
